vi "MessageQueue_PreviewAllQueueElements.vi"(0 "QueueIn":refnum<queue>, 3 "FlushElements":bool, 5 "ErrorIn":errorcluster) -> (14 "QueueOut":refnum<queue>, 16 "ElemtentInQueue":T1[](array[typedef]), 17 "NoOfElementsInQueue":i32, 19 "ErrorOut":errorcluster)   [LabVIEW 2016]
doc: "Zeigt die im Queue vorhandenen Elemente. Flush Queue leert den Queue.\n\nsige / 4.12.13"
uses:
  private/MessageQueue.MessageTypeDef.ctl
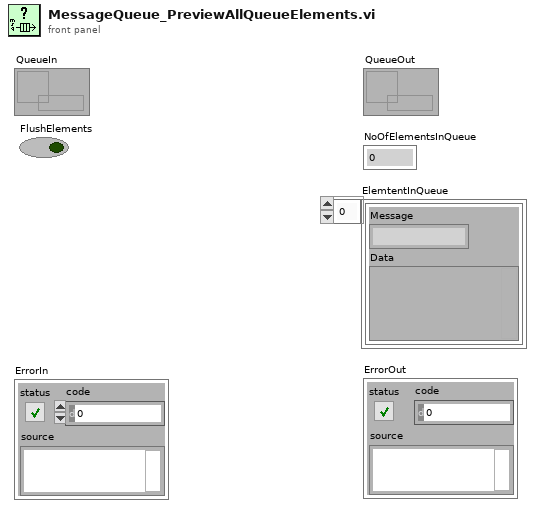
[diagram p1: front panel]
types:
  T1 = typedef "MessageQueue.MessageTypeDef.ctl" = cluster{"Message":string, "Data":variant}
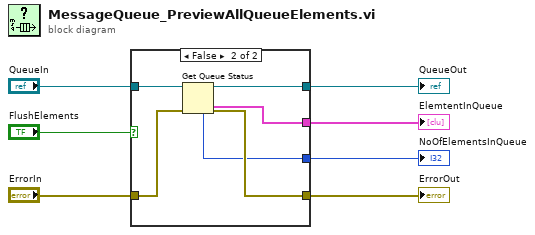
[diagram p0: block diagram]
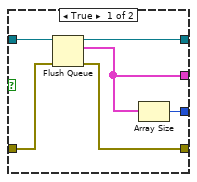
[diagram p2: hidden frame]
diagram:
  n1 = case shown="False" "FlushElements" {
    tunnel: "QueueIn" -> [w13 w19]
    tunnel: [w10 w18] -> w6
    tunnel: [w12 w17] -> w5
    tunnel: "ErrorIn" -> [w11 w16]
    tunnel: [w8 w15] -> w3
    tunnel: [w9 w14] -> w2
    frame True {
      n2 = Flush Queue(queue=w13, error in (no error)=w11) -> (queue out=w12:refnum<queue>, remaining elements=w8:T1[], error out=w10:errorcluster)
      n3 = Array Size(array=w8) -> (size(s)=w9:i32)
    }
    frame False {
      n4 = Get Queue Status(queue=w19, error in (no error)=w16) -> (queue out=w17:refnum<queue>, error out=w18:errorcluster, # elements in queue=w14:i32, elements=w15:T1[])  [unwired: 1 in, 4 out]
    }
  }
  "ErrorOut" <- w6
  "QueueOut" <- w5
  "ElemtentInQueue" <- w3
  "NoOfElementsInQueue" <- w2
